vi "SR430_get_trig_offset.vi"(0 "address":T1, 5 "error in (no error)":errorcluster) -> (14 "address out":T1, 16 "triggerOffset":i32, 19 "error out":errorcluster)   [LabVIEW 2009, in "SR430Driver.lvlib"]
doc: "Gets the Trigger Offset from the device.\n\nThe Offset value can go from 0 to 16384 per step of 16.\n\nVI Tree for the SR430 Multi-Channel Scaler from Staford Research Systems.\n\nHistory: 24-APR-2002, Dietrich Beck\n\nCopyright (C)\nGesellschaft für Schwerionenforschung, GSI\nPlanckstr. 1\n64291 Darmstadt\nGermany\n\nContact: D.Beck@gsi.de \n\nThis program is free software; you can redistribute it and/or modify it under the terms of the \nGNU General Public License as published by the Free Software Foundation; either version 2 of the license, or (at your option) any later version.\n\nThis program is distributed in the hope that it will be useful, but WITHOUT ANY WARRANTY; without even the implied warranty of MERCHANTABILITY or FITNESS FOR A PARTICULAR PURPOSE. See the GNU General License for more details (http://www.gnu.org).\n\nGesellschaft für Schwerionenforschung, GSI\nPlanckstr. 1, 64291 Darmstadt, Germany\nFor all questions and ideas contact: M.Richter@gsi.de, K.Poppensieker, H.Brand@gsi.de or D.Beck@gsi.de.\nLast update: 11-APR-2002"
uses:
  SR430Driver.lvlib
  SR430_VISA Control.ctl
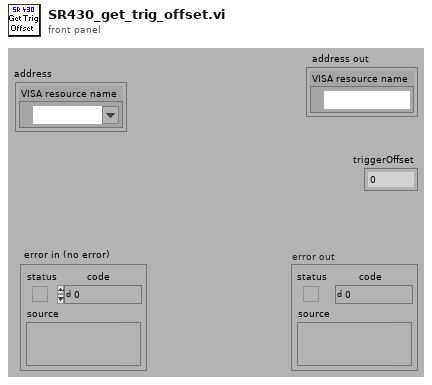
[diagram p1: front panel]
types:
  T1 = typedef "SR430Driver.lvlib/SR430_VISA Control.ctl" = cluster{"VISA resource name":refnum<visa-resource-name>}
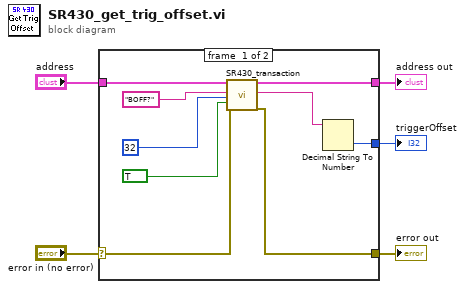
[diagram p0: block diagram]
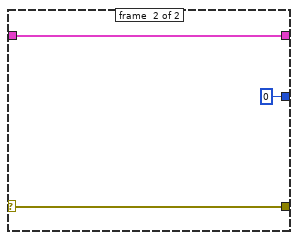
[diagram p2: hidden frame]
diagram:
  n1 = case shown="No Error" "error in (no error)" {
    selector: "error in (no error)" -> [w6 w15]
    tunnel: [w14 0] -> w5
    tunnel: [w12 w15] -> w4
    tunnel: [w11 w17] -> w3
    tunnel: "address" -> [w10 w17]
    frame #0 {
      n2 = call "SR430_transaction.vi"("SR430 VISA Cluster"=w10, "SR430 Command String"="BOFF?" ("write buffer"), "Bytes to read (1024)"=32 ("byte count"), "Read (FALSE)"=TRUE, "error in (no error)"=w6) -> ("dup SR430 VISA Cluster"=w11:T1, "SR430 Response"=w13:string, "error out"=w12:errorcluster)  [unwired: 11 in, 1 out]
      n3 = Decimal String To Number(string=w13) -> (number=w14:i32)  [unwired: 2 in, 1 out]
    }
    frame #1 {
    }
  }
  "error out" <- w4
  "triggerOffset" <- w5
  "address out" <- w3
